vi "Close.vi"(8 "error in (no error)":errorcluster, 11 "VISA resource name":refnum<visa-resource-name>) -> (0 "error out":errorcluster)   [LabVIEW 2020, in "Rohde&Schwarz CMP LR WPAN Measurement.lvlib"]
doc: "This VI performs the following operations:\n- Closes the instrument VISA session.\n- Destroys the instrument driver session and all of its properties.\n\nNote:\n- After calling <b>Close.vi</b>, you cannot use any of the instrument driver VIs until you call <b>Initialize.vi</b>"
uses:
  <instrlib>/Rohde&Schwarz CMP LR WPAN Measurement/Rohde&Schwarz CMP LR WPAN Measurement.lvlib
  <instrlib>/Rohde&Schwarz CMP LR WPAN Measurement/Private/rsidr_core.llb/rsidr_core.lvlib
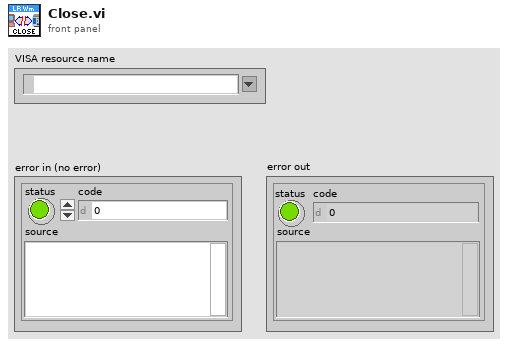
[diagram p1: front panel]
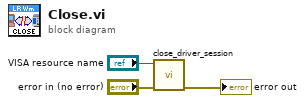
[diagram p0: block diagram]
diagram:
  n1 = call <instrlib>:"close_driver_session.vi"("error in"="error in (no error)", "VISA resource name"="VISA resource name") -> ("error out"=→"error out":errorcluster)  [unwired: 9 in]
